vi "act-0020-1-cor.vi"() -> ()   [LabVIEW 2010]
uses:
  lv_07/lv_07.lvlib
panel:
  out "Cc init":dbl
  out "T init":dbl
  out "Ccpc nv":dbl
  in  "Cc":dbl
  in  "T":dbl
  in  "Ccpc anc":dbl
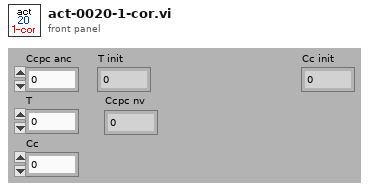
[diagram p1: front panel]
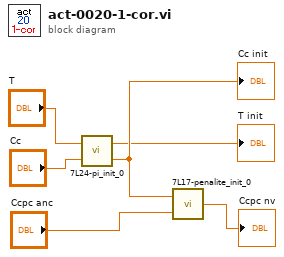
[diagram p0: block diagram]
diagram:
  n1 = call "7L24-pi_init_0.vi"("Cc"="Cc", "T"="T") -> ("Cc init"=w6:dbl, "T init"=→"T init":dbl)
  "Cc init" <- w6
  n2 = call "7L17-penalite_init_0.vi"("Ccpc"="Ccpc anc", "Cc"=w6) -> ("Ccpc init"=→"Ccpc nv":dbl)
